vi "ConfigFreqVoltRange.vi"(8 "error in (no error)":errorcluster, 11 "HP3458aDMM in":refnum<class "HP3458aDMM.lvclass">) -> (0 "error out":errorcluster, 3 "HP3458aDMM out":refnum<class "HP3458aDMM.lvclass">)   [LabVIEW 2014, in "SamplerPlugins.lvlib" / "HP3458aDMM.lvclass"]
uses:
  HP3458aDMM.lvclass
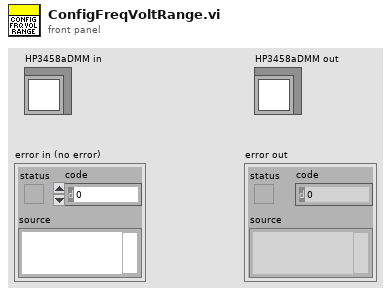
[diagram p1: front panel]
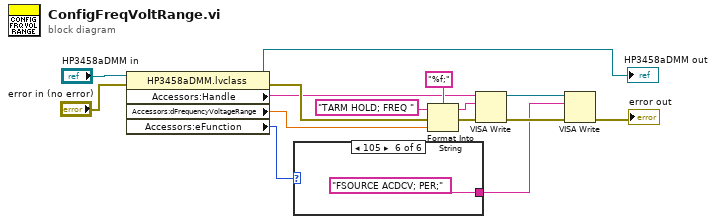
[diagram p0: block diagram]
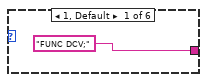
[diagram p2: hidden frame]
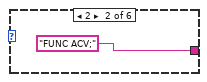
[diagram p3: hidden frame]
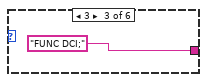
[diagram p4: hidden frame]
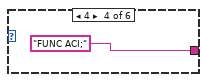
[diagram p5: hidden frame]
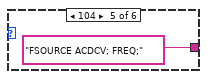
[diagram p6: hidden frame]
diagram:
  n1 = property class="HP3458aDMM.lvclass"(reference="HP3458aDMM in", error in="error in (no error)") -> (reference out=→"HP3458aDMM out":refnum<class "HP3458aDMM.lvclass">, error out=w12:errorcluster, "Accessors:Handle"=w7:string, "Accessors:dFrequencyVoltageRange"=w11:dbl, "Accessors:eFunction"=w5:u16)
  n2 = case shown="105" w5 {
    tunnel: ["FUNC DCV;" "FUNC ACV;" "FUNC DCI;" "FUNC ACI;" "FSOURCE ACDCV; FREQ;" "FSOURCE ACDCV; PER;"] -> w2
    frame 1, Default {
    }
    frame 2 {
    }
    frame 3 {
    }
    frame 4 {
    }
    frame 104 {
    }
    frame 105 {
    }
  }
  n3 = Format Into String(format string="%f;", initial string="TARM HOLD; FREQ ", error in=w12, w11) -> (resulting string=w6:string, error out=w8:errorcluster)
  n4 = VISA Write(VISA resource name=w7, write buffer=w6, error in (no error)=w8) -> (VISA resource name out=w1:refnum<visa-resource-name>, error out=w4:errorcluster)  [unwired: 1 out]
  n5 = VISA Write(VISA resource name=w1, write buffer=w2, error in (no error)=w4) -> (error out=→"error out":errorcluster)  [unwired: 2 out]
